vi "rs3 get device extrinsics3.vi"(8 "error in (no error)":errorcluster, 10 "Target Stream Profile":u64=338256128, 11 "Origin Stream Profile":u64=338256128) -> (0 "error out":errorcluster, 2 "error":u64, 5 "extrin out":T1={"rotation[0]"=1.0, "rotation[1]"=0.0, "rotation[2]"=0.0, "rotation[3]"=0.0, "rotation[4]"=1.0, "rotation[5]"=0.0, "rotation[6]"=0.0, "rotation[7]"=0.0, "rotation[8]"=1.0, "translation[0]"=-0.053904004, "translation[1]"=0.0, "translation[2]"=0.0})   [LabVIEW 2017, in "libRealSense3.lvlib"]
doc: "Provides all the sensor extrinsics, such as the distance (i.e. baseline) between two sensors. Note that you need to select the streams. \nFor example: if you want to know the baseline of a stereo module you will need to enter the HANDLES (profile) for the Left and Right streams here."
uses:
  libRealSense3.lvlib
  realsense2.dll
panel:
  # "RS3 Get Device Extrinsics 4"
  # "(C) Intel Corp. 2017,  AGJ"
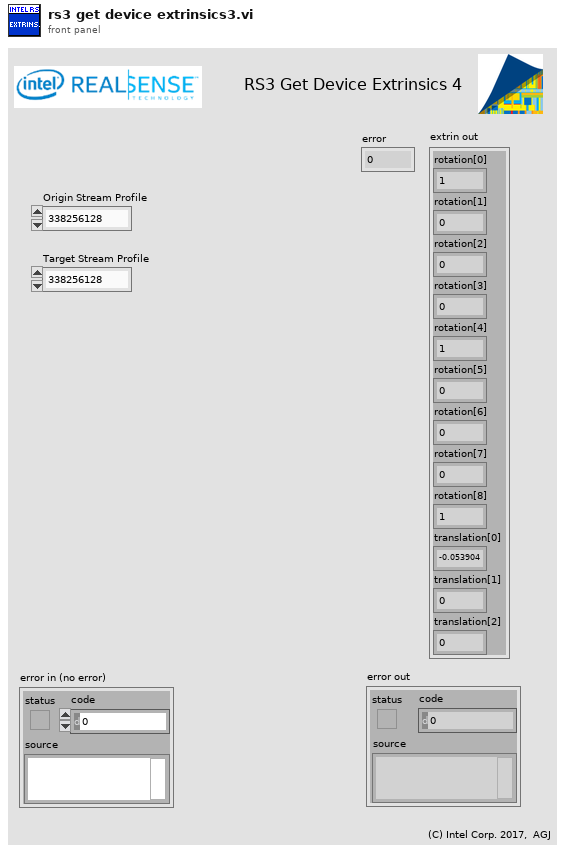
[diagram p1: front panel]
types:
  T1 = cluster{"rotation[0]":sgl, "rotation[1]":sgl, "rotation[2]":sgl, "rotation[3]":sgl, "rotation[4]":sgl, "rotation[5]":sgl, "rotation[6]":sgl, "rotation[7]":sgl, "rotation[8]":sgl, "translation[0]":sgl, "translation[1]":sgl, "translation[2]":sgl}
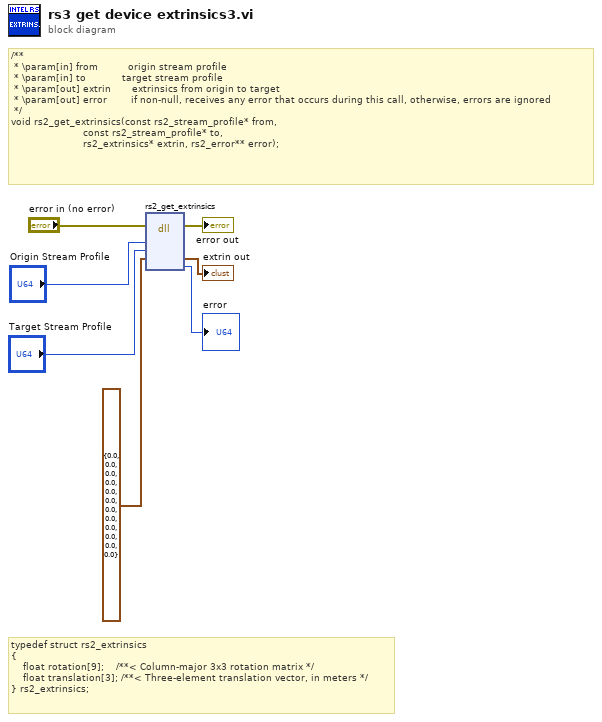
[diagram p0: block diagram]
diagram:
  # "typedef struct rs2_extrinsics\n{\n    float rotation[9];    /**< Column-major 3x3 rotation matrix */\n    float translation[3]; /**< Three-element translation vector, in meters */\n} rs2_extrinsics;"
  # "/**\n * \\param[in] from          origin stream profile\n * \\param[in] to            target stream profile\n * \\param[out] extrin       extrinsics from origin to target\n * \\param[out] error        if non-null, receives any error that occurs during this call, otherwise, errors are ignored\n */\nvoid rs2_get_extrinsics(const rs2_stream_profile* from,\n                        const rs2_stream_profile* to,\n                        rs2_extrinsics* extrin, rs2_error** error);"
  n1 = dll-call lib="C:/Users/agrunnet/Documents/libRealSense6/realsense2.dll" fn="rs2_get_extrinsics"(error in="error in (no error)", "Origin stream"="Origin Stream Profile", "Target stream"="Target Stream Profile", "extrin"=T1 {"rotation[0]"=0.0, "rotation[1]"=0.0, "rotation[2]"=0.0, "rotation[3]"=0.0, "rotation[4]"=0.0, "rotation[5]"=0.0, "rotation[6]"=0.0, "rotation[7]"=0.0, "rotation[8]"=0.0, "translation[0]"=0.0, "translation[1]"=0.0, "translation[2]"=0.0}) -> (error out=→"error out":errorcluster, "extrin"=→"extrin out":T1, "error"=→"error":u64)  [unwired: 6 in, 1 out]
